vi "运维调试_五参数.vi"() -> ()   [LabVIEW 2016, in "斯坦道仪器.lvlib"]
uses:
  <vilib>/Utility/miscctls.llb/LVPointTypeDef.ctl
  <vilib>/Utility/config.llb/NI_LVConfig.lvlib
panel:
  in  "质控参数设置":bool
  in  "打开串口":bool
  in  "释放串口":bool
  out "多参数横条运行状态":T1(xcontrol)
  in  "数据区":i32(listbox)
  in  "探头选择":u16(ring)=9 items=["氨氮"=3, "水温"=9, "pH值"=10, "溶解氧"=11, "电导率"=12, "浊度"=13, "叶绿素a"=14, "藻密度"=15, "蓝绿藻"=16, "氧化还原电位"=17, "溶解氧%"=18, "盐度"=19]
  in  "测量数据区读取":bool
  in  "测量数据区":i32(listbox)
  in  "状态告警区读取":bool
  in  "状态告警区":i32(listbox)
  in  "读取KB":bool
  in  "写入KB":bool
  out "B":dbl caption="校准值B:"
  out "K":dbl caption="校准值K:"
  in  "校准区探头选择":u16(ring)=9 items=["氨氮"=3, "水温"=9, "pH值"=10, "溶解氧"=11, "电导率"=12, "浊度"=13, "叶绿素a"=14, "藻密度"=15, "蓝绿藻"=16, "氧化还原电位"=17, "溶解氧%"=18, "盐度"=19]
  in  "停止测量(单探)":bool
  in  "启动测量(单探)":bool
  in  "控制命令区探头选择":u16(ring)=9 items=["氨氮"=3, "水温"=9, "pH值"=10, "溶解氧"=11, "电导率"=12, "浊度"=13, "叶绿素a"=14, "藻密度"=15, "蓝绿藻"=16, "氧化还原电位"=17, "溶解氧%"=18, "盐度"=19]
  in  "同步时间":bool
  in  "初始化(清洗)":bool
  in  "停止测量(全部)":bool
  in  "启动测量(全部)":bool
  in  "关键参数区读取":bool
  in  "关键参数区":i32(listbox)
  in  "传感器参数读取":bool
  in  "传感器区":i32(listbox)
  in  "返回":bool
  in  "设置":bool
  out "运行状态":string
  out "开机状态":bool
  in  "停止":bool
  in  "手动启动":bool
  out "集成报警信息":string
  # "控制命令区"
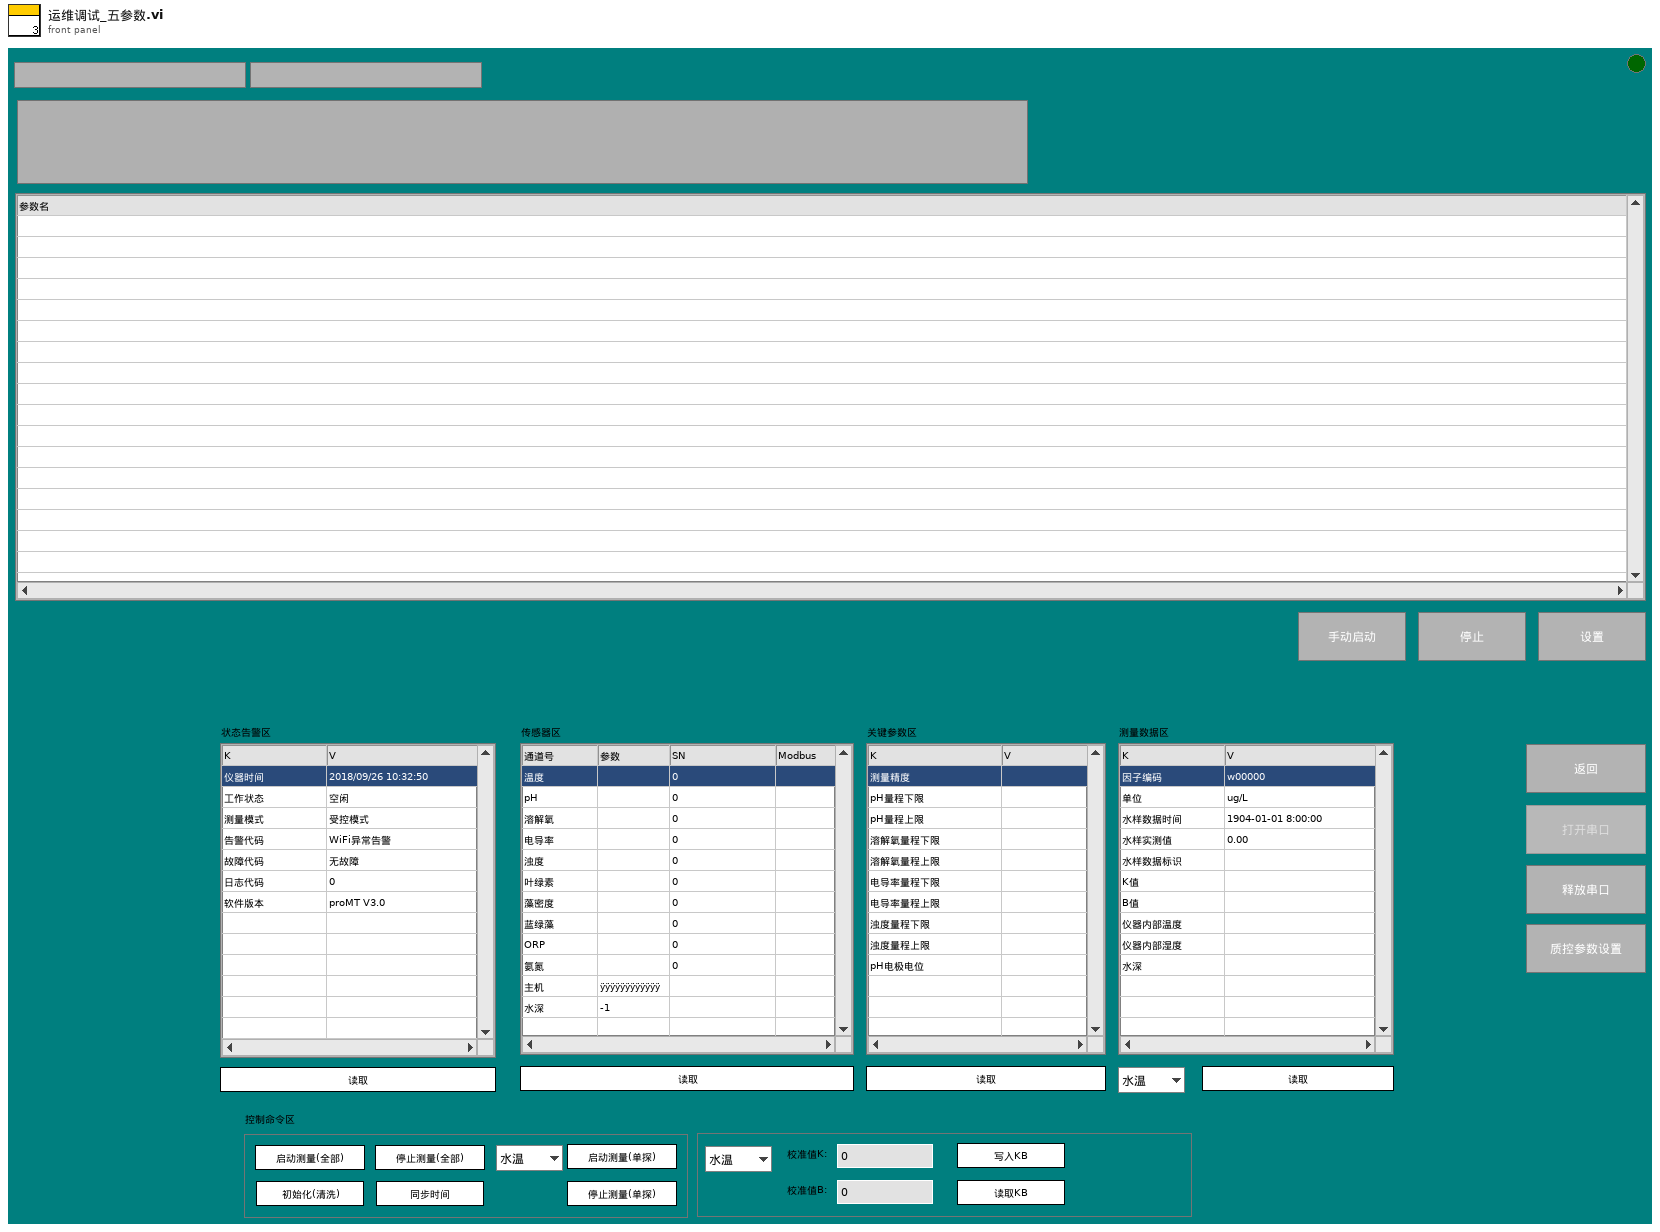
[diagram p1: front panel]
types:
  T1 = cluster{"系统时间":timestamp, "工作状态":u16, "测量模式":u16, "告警代码":enum16{"无告警", "缺试剂告警", "缺水样告警", "缺蒸馏水告警", "缺标液告警", "仪表漏液告警", "标定异常告警", "超量程告警", "加热异常", "低试剂预警", "超上限告警", "超下限告警", "仪表内部其他异常", "滴定异常告警", "电极异常告警", "量程切换告警", "参数设置告警", "PH电极电位异常", "电导率电极异常", "浊度光度异常", "溶解氧电极异常", "溶解氧光强异常", "温度异常告警", "PH异常告警", "溶解氧异常告警", "电导率异常告警", "浊度异常告警", "叶绿素异常告警", "藻密度异常告警", "蓝绿藻异常告警", "ORP异常告警", "氨氮异常告警", "清洁刷异常告警", "SD卡异常告警", "蓝牙异常告警", "Wifi异常告警", "流程异常告警"}, "故障代码":enum16{"无故障", "电机故障", "温度故障", "通讯故障", "滴定故障"}, "日志代码":u16, "软件版本":string}
  T2 = typedef "LVPointTypeDef.ctl" = cluster{"Horizontal":i16, "Vertical":i16}
  T3 = cluster{"时间标识":timestamp, "设备":string, "日志信息":string}
  T4 = enum16{"无告警", "缺试剂告警", "缺水样告警", "缺蒸馏水告警", "缺标液告警", "仪表漏液告警", "标定异常告警", "超量程告警", "加热异常", "低试剂预警", "超上限告警", "超下限告警", "仪表内部其他异常", "滴定异常告警", "电极异常告警", "量程切换告警", "参数设置告警", "PH电极电位异常", "电导率电极异常", "浊度光度异常", "溶解氧电极异常", "溶解氧光强异常", "温度异常告警", "PH异常告警", "溶解氧异常告警", "电导率异常告警", "浊度异常告警", "叶绿素异常告警", "藻密度异常告警", "蓝绿藻异常告警", "ORP异常告警", "氨氮异常告警", "清洁刷异常告警", "SD卡异常告警", "蓝牙异常告警", "Wifi异常告警", "流程异常告警"}
  T5 = cluster{"水温":dbl, "pH":dbl, "DO":dbl, "Cond":dbl, "Turb":dbl, "叶绿素":dbl, "藻密度":dbl, "蓝绿藻":dbl, "ORP":dbl, "NH3N":dbl}
  T6 = cluster{"因子编码":string, "单位":string, "标样参考值":sgl, "水样数据时间":timestamp, "水样实测值":sgl, "水样数据标识":string, "K":sgl, "B":sgl, "T":sgl, "H":sgl, "水深":sgl, "探头温度":sgl}
  T7 = typedef "NI_LVConfig.lvlib/Config Data RefNum.ctl" = refnum<k1>
  T8 = enum8{"Enabled", "Disabled", "Disabled and Grayed Out"}
  T9 = cluster{"测量模式":enum16{"待机", "水样测试", "标样核查", "零点核查", "跨度核查", "空白测试", "平行样测试", "加标回收", "空白校准", "标样校准", "初始化（清洗）"}, "数据标记表":string, "测量时间":dbl}
  T10 = cluster{"水温标准液标准浓度":dbl, "酸碱度标准液标准浓度":dbl, "溶解氧标准液标准浓度":dbl, "电导率标准液标准浓度":dbl, "浊度标准液标准浓度":dbl}
  T11 = cluster{"确定":bool, "水温标准液标准浓度":dbl, "酸碱度标准液标准浓度":dbl, "溶解氧标准液标准浓度":dbl, "电导率标准液标准浓度":dbl, "浊度标准液标准浓度":dbl}
  T12 = enum32{"Bad", "Idle", "Run top level", "Running"}
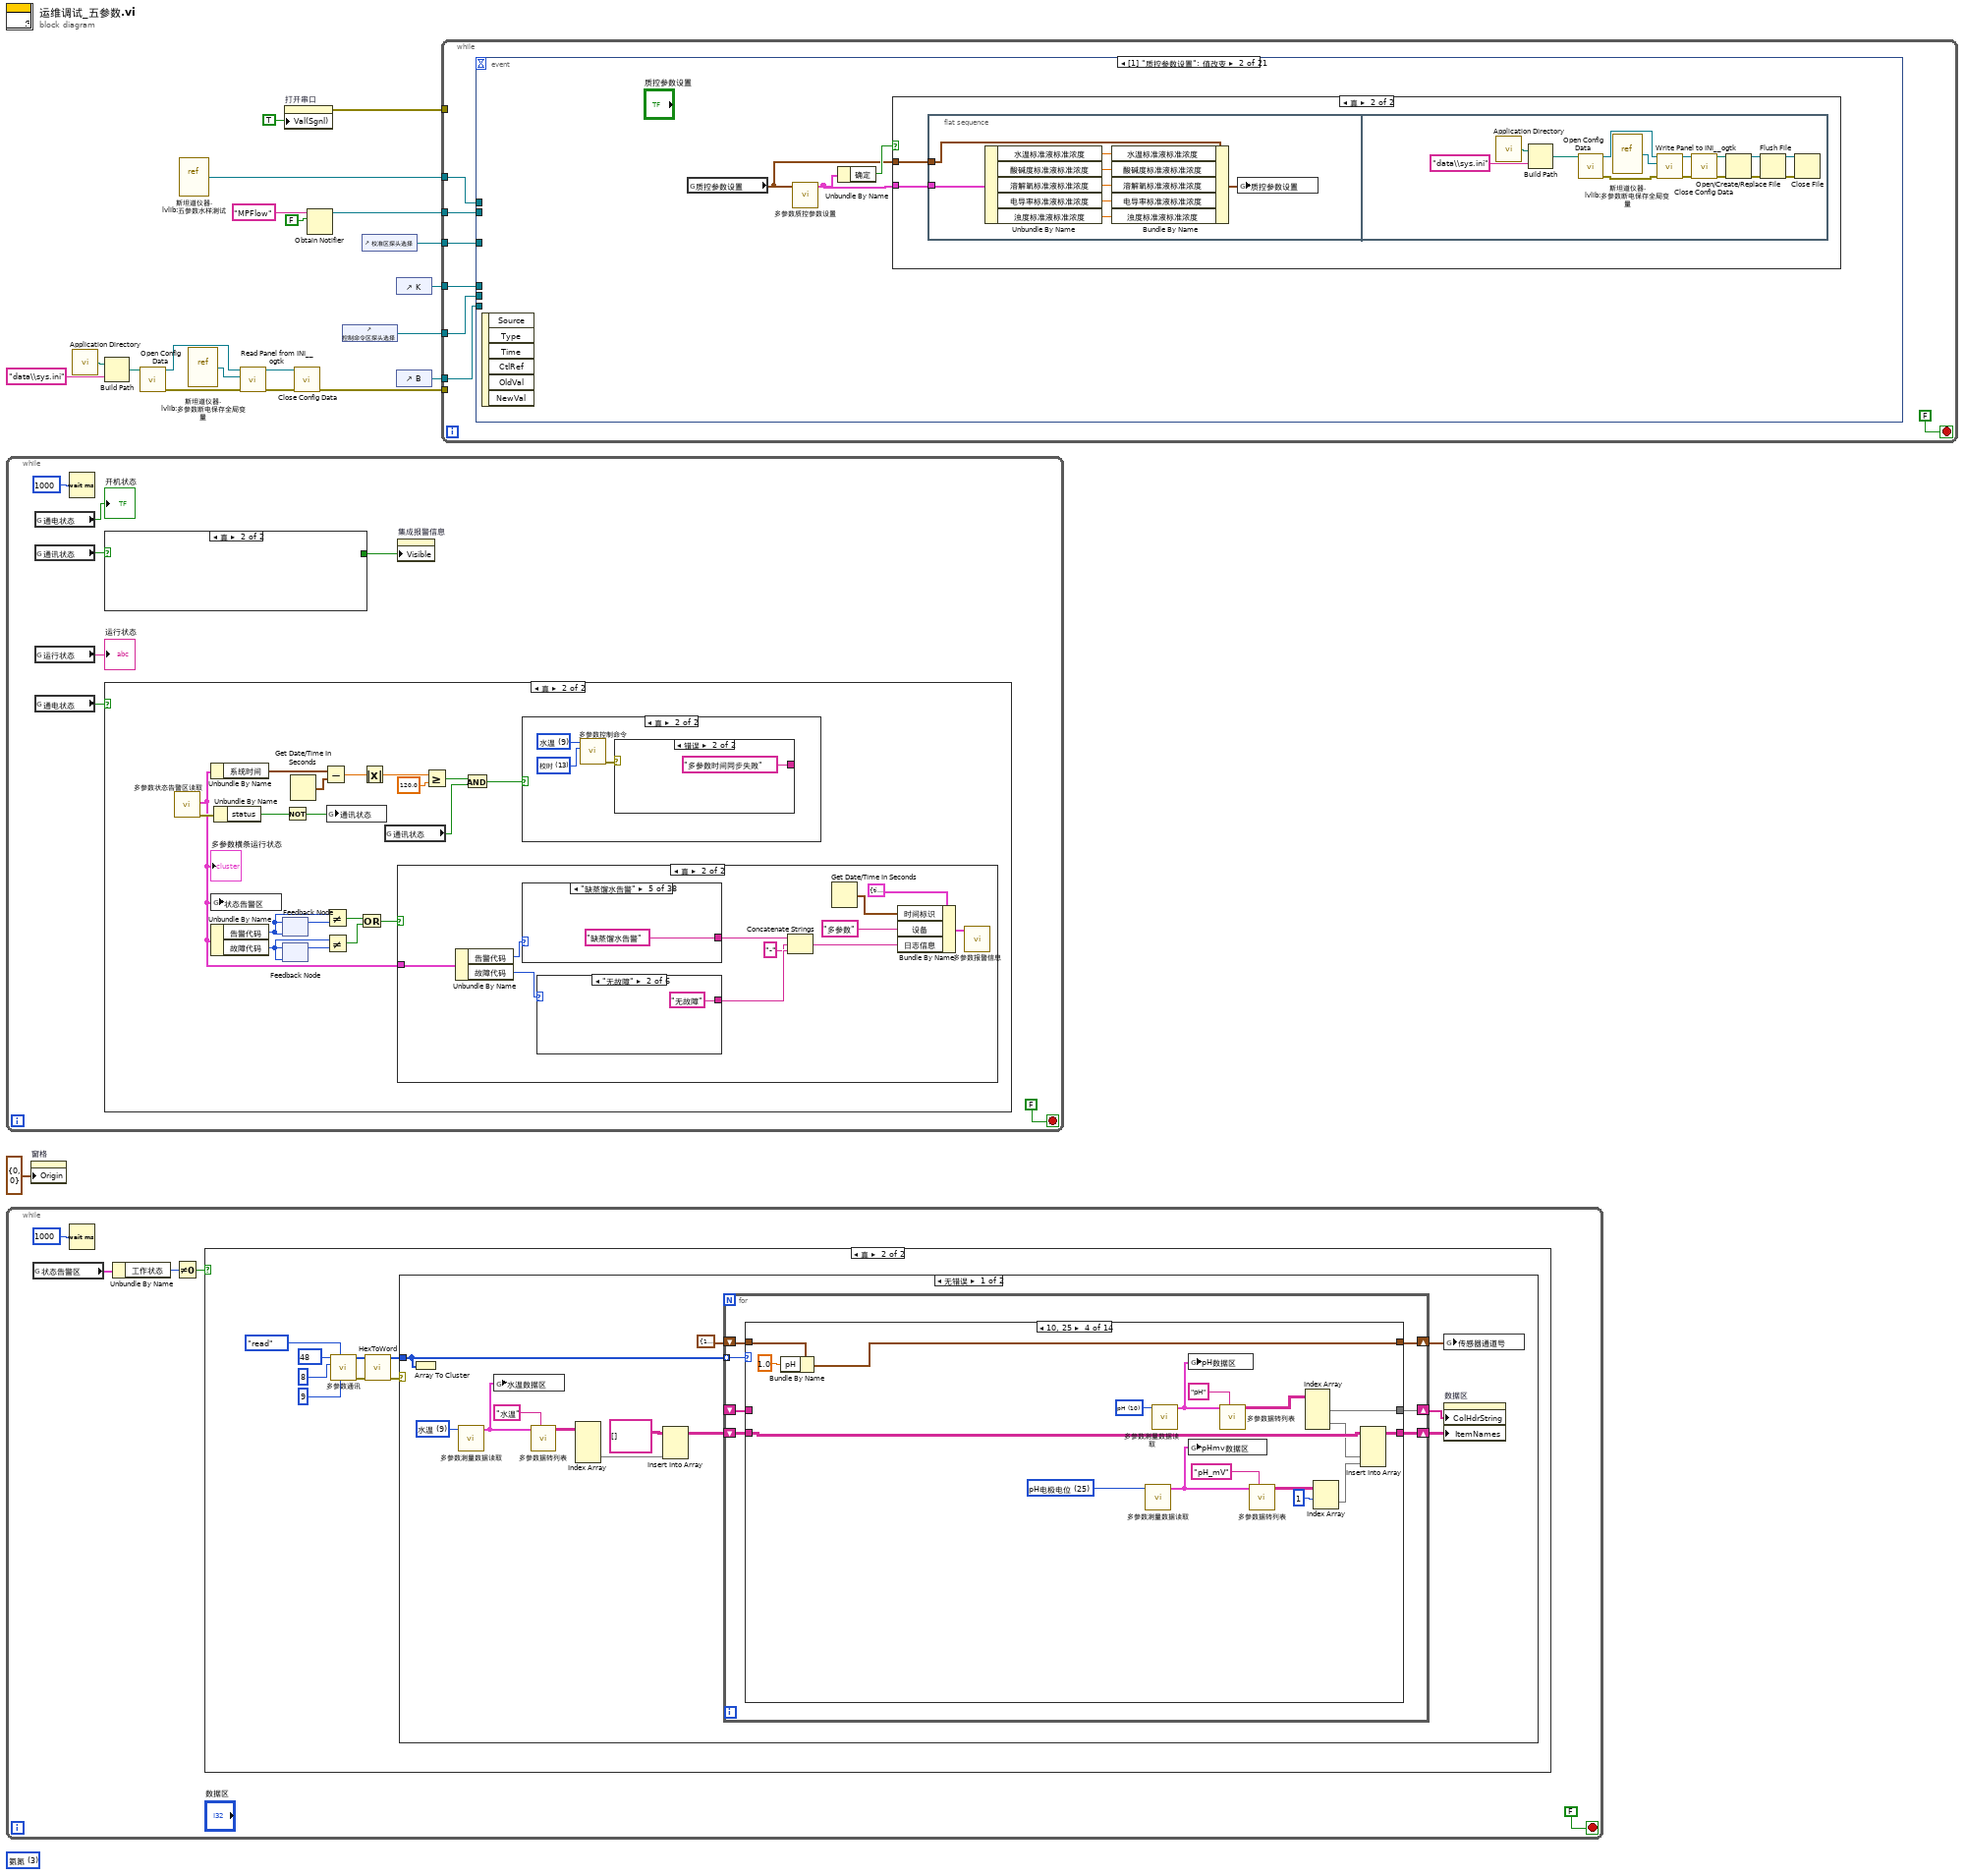
[diagram p0: block diagram]
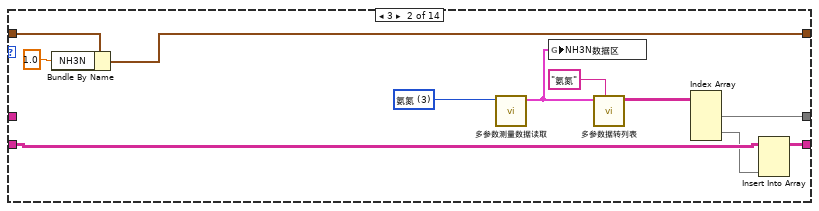
[diagram p4: hidden frame]
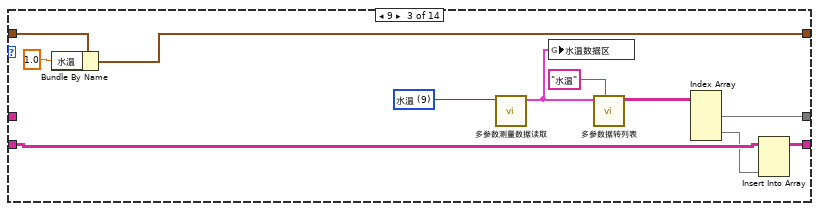
[diagram p5: hidden frame]
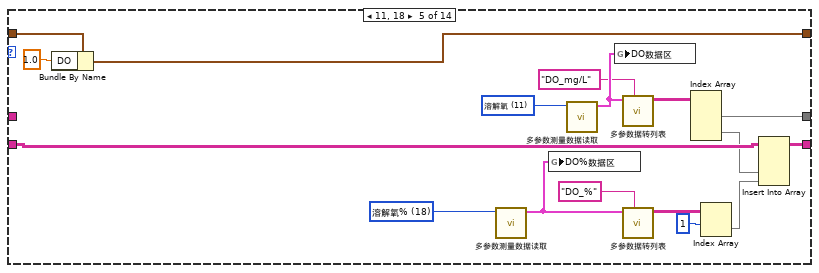
[diagram p6: hidden frame]
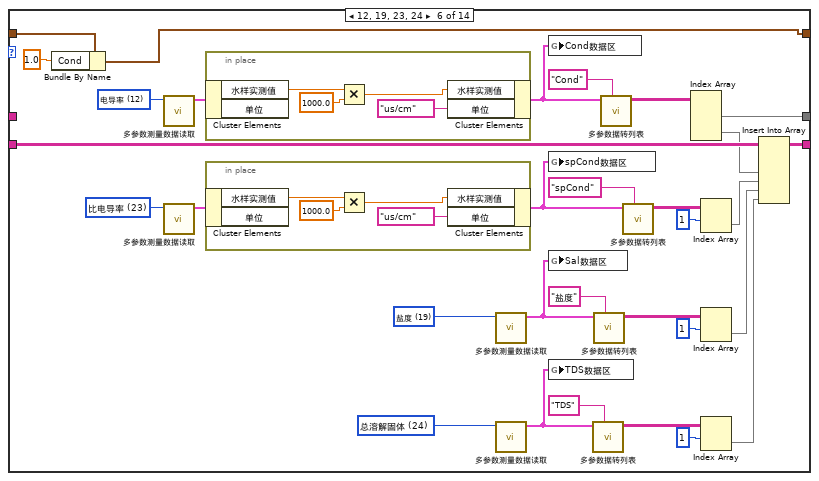
[diagram p7: hidden frame]
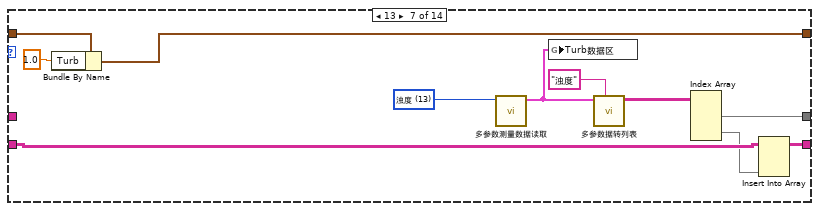
[diagram p8: hidden frame]
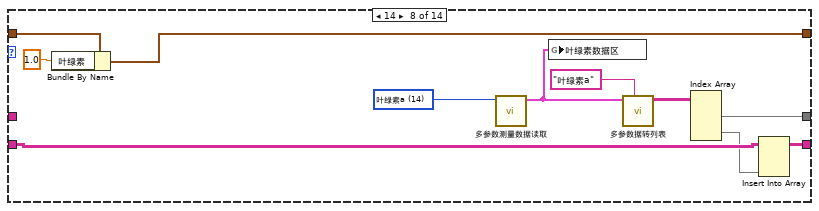
[diagram p9: hidden frame]
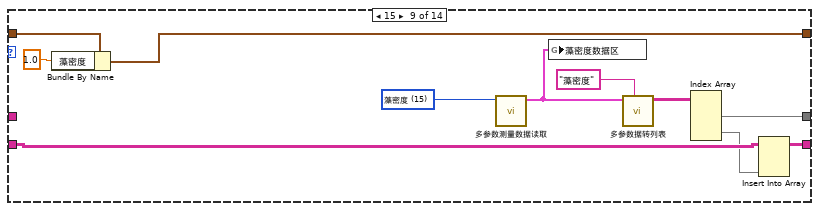
[diagram p10: hidden frame]
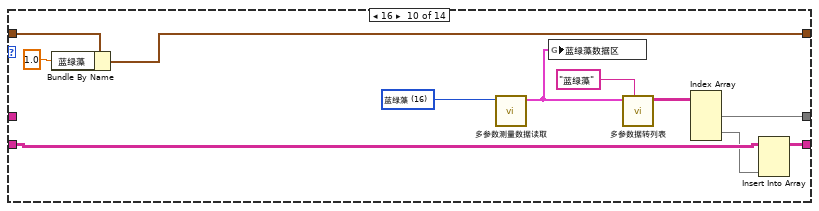
[diagram p11: hidden frame]
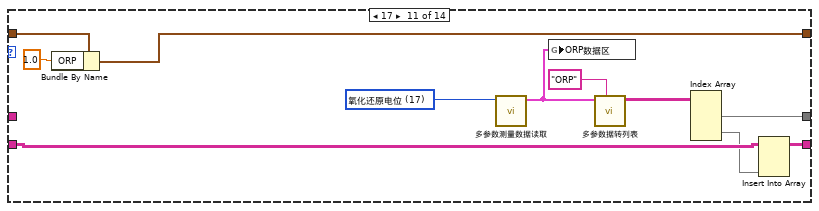
[diagram p12: hidden frame]
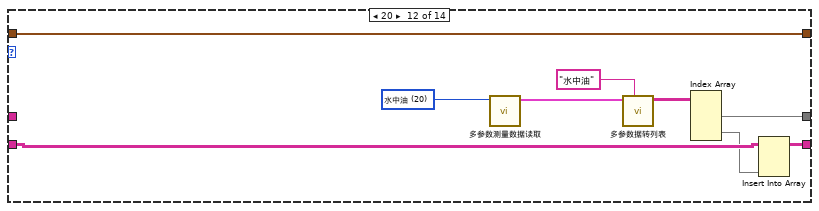
[diagram p13: hidden frame]
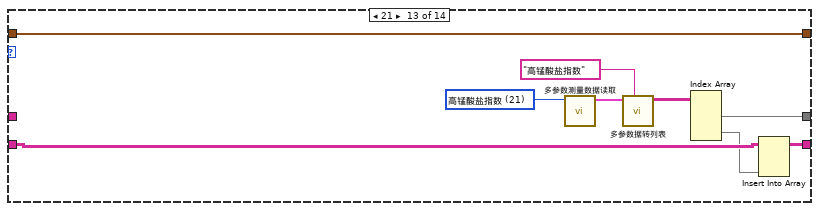
[diagram p14: hidden frame]
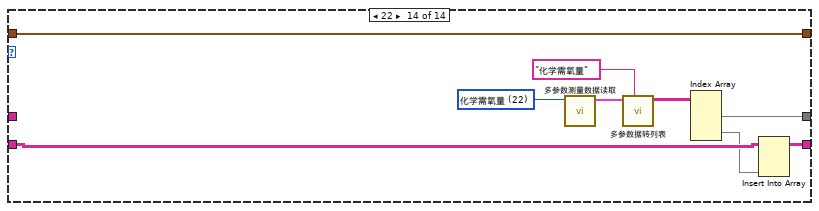
[diagram p15: hidden frame]
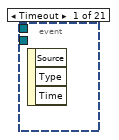
[diagram p17: hidden frame]
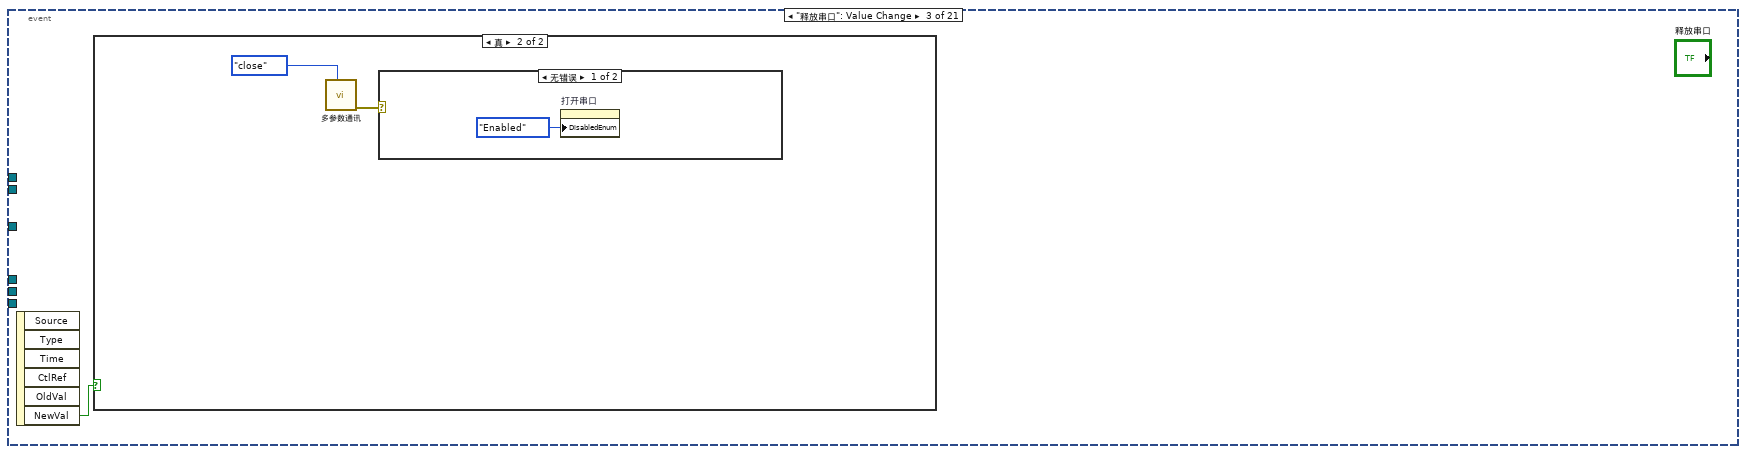
[diagram p19: hidden frame]
diagram:
  (unwired) u16 3 items=["氨氮"=3, "水温"=9, "pH"=10, "溶解氧"=11, "电导率"=12, "浊度"=13, "叶绿素a"=14, "藻密度"=15, "蓝绿藻"=16, "氧化还原电位"=17, "溶解氧%"=18, "盐度"=19, "水中油"=20, "高锰酸盐指数"=21, "化学需氧量"=22, "比电导率"=23, "总溶解固体"=24, "pH电极电位"=25] ("下拉列表")
  n1 = while {
    stop <- FALSE stop-if-true
    n2 = global read "多参数全局变量.vi" "通电状态"() -> (→"开机状态":bool)
    n3 = global read "多参数全局变量.vi" "通讯状态"() -> (w25:bool)
    n4 = global read "多参数全局变量.vi" "运行状态"() -> (→"运行状态":string)
    n5 = global read "多参数全局变量.vi" "通电状态"() -> (w21:bool)
    n6 = Wait (ms)(milliseconds to wait=u32 1000 ("等待时间（毫秒）")) -> ()  [unwired: 1 out]
    n7 = case shown="真" w25 {
      tunnel: [TRUE ("可见") _] -> w24
      frame False {
        "集成报警信息" <- "通讯异常" ("集成报警信息")
      }
      frame True {
      }
    }
    n8 = case shown="真" w21 {
      frame False {
      }
      frame True {
        n9 = call "多参数状态告警区读取.vi"() -> ("error out"=w39:errorcluster, "状态告警块"=w36:T1)  [unwired: 9 in, 1 out]
        "多参数横条运行状态" <- w36
        n10 = Unbundle By Name(w36) -> ("系统时间"=w35:timestamp)
        n11 = global write "多参数全局变量.vi" "状态告警区"(w36) -> ()
        n12 = Unbundle By Name(w36) -> ("告警代码"=w45:T4, "故障代码"=w43:enum16{"无故障", "电机故障", "温度故障", "通讯故障", "滴定故障"})
        n13 = Unbundle By Name(w39) -> ("status"=w38:bool)
        n14 = feedback #1(w45) -> (w46:T4)
        n15 = feedback-in #1(w45) -> ()
        n16 = feedback #2(w43) -> (w44:enum16{"无故障", "电机故障", "温度故障", "通讯故障", "滴定故障"})
        n17 = feedback-in #2(w43) -> ()
        n18 = Not(x=w38) -> (.not. x?=w37:bool)
        n19 = Get Date/Time In Seconds() -> (seconds since 1Jan1904=w34:timestamp)
        n20 = Subtract(x=w35, y=w34) -> (x-y=w33:dbl)
        n21 = Not Equal?(x=w45, y=w46) -> (x != y?=w41:bool)
        n22 = Not Equal?(x=w43, y=w44) -> (x != y?=w42:bool)
        n23 = global write "多参数全局变量.vi" "通讯状态"(w37) -> ()
        n24 = Or(x=w41, y=w42) -> (x .or. y?=w40:bool)
        n25 = Absolute Value(x=w33) -> (abs(x)=w32:dbl)
        n26 = global read "多参数全局变量.vi" "通讯状态"() -> (w28:bool)
        n27 = case shown="真" w40 {
          tunnel: w36 -> [_ w62]
          frame False {
          }
          frame True {
            n28 = Unbundle By Name(w62) -> ("告警代码"=w61:T4, "故障代码"=w60:enum16{"无故障", "电机故障", "温度故障", "通讯故障", "滴定故障"})
            n29 = case shown="\"缺蒸馏水告警\"" w61 {
              selector: w61 -> [w73 _ _ _ _ _ _ _ _ _ _ _ _ _ _ _ _ _ _ _ _ _ _ _ _ _ _ _ _ _ _ _ _ _ _ _ _ _]
              tunnel: [w72 "无告警" "缺试剂告警" "缺水样告警" "缺蒸馏水告警" "缺标液告警" "仪表漏液告警" "标定异常告警" "超量程告警" "加热异常" "低试剂预警" "超上限告警" "超下限告警" "仪表内部其他异常" "滴定异常告警" "电极异常告警" "量程切换告警" "参数设置告警" "PH电极电位异常" "电导率电极异常" "浊度光度异常" "溶解氧电极异常" "溶解氧光强异常" "温度异常告警" "PH异常告警" "溶解氧异常告警" "电导率异常告警" "浊度异常告警" "叶绿素异常告警" "藻密度异常告警" "蓝绿藻异常告警" "ORP异常告警" "氨氮异常告警" "清洁刷异常告警" "SD卡异常告警" "蓝牙异常告警" "WiFi异常告警" "流程异常告警"] -> w59
              frame Default {
                n30 = Format Into String(format string="%d" ("格式字符串"), initial string="未知" ("工作状态"), w73) -> (resulting string=w72:string)  [unwired: 1 in, 1 out]
              }
              frame "无告警" {
              }
              frame "缺试剂告警" {
              }
              frame "缺水样告警" {
              }
              frame "缺蒸馏水告警" {
              }
              frame "缺标液告警" {
              }
              frame "仪表漏液告警" {
              }
              frame "标定异常告警" {
              }
              frame "超量程告警" {
              }
              frame "加热异常" {
              }
              frame "低试剂预警" {
              }
              frame "超上限告警" {
              }
              frame "超下限告警" {
              }
              frame "仪表内部其他异常" {
              }
              frame "滴定异常告警" {
              }
              frame "电极异常告警" {
              }
              frame "量程切换告警" {
              }
              frame "参数设置告警" {
              }
              frame "PH电极电位异常" {
              }
              frame "电导率电极异常" {
              }
              frame "浊度光度异常" {
              }
              frame "溶解氧电极异常" {
              }
              frame "溶解氧光强异常" {
              }
              frame "温度异常告警" {
              }
              frame "PH异常告警" {
              }
              frame "溶解氧异常告警" {
              }
              frame "电导率异常告警" {
              }
              frame "浊度异常告警" {
              }
              frame "叶绿素异常告警" {
              }
              frame "藻密度异常告警" {
              }
              frame "蓝绿藻异常告警" {
              }
              frame "ORP异常告警" {
              }
              frame "氨氮异常告警" {
              }
              frame "清洁刷异常告警" {
              }
              frame "SD卡异常告警" {
              }
              frame "蓝牙异常告警" {
              }
              frame "Wifi异常告警" {
              }
              frame "流程异常告警" {
              }
            }
            n31 = case shown="\"无故障\"" w60 {
              selector: w60 -> [w64 _ _ _ _ _]
              tunnel: [w63 "无故障" "电机故障" "温度故障" "通讯故障" "滴定故障"] -> w58
              frame Default {
                n32 = Format Into String(format string="%d" ("格式字符串"), initial string="未知" ("工作状态"), w64) -> (resulting string=w63:string)  [unwired: 1 in, 1 out]
              }
              frame "无故障" {
              }
              frame "电机故障" {
              }
              frame "温度故障" {
              }
              frame "通讯故障" {
              }
              frame "滴定故障" {
              }
            }
            n33 = Concatenate Strings(w59, "-" ("字符串"), w58) -> (w54:string)
            n34 = Get Date/Time In Seconds() -> (seconds since 1Jan1904=w53:timestamp)
            n35 = Bundle By Name(cluster=T3 {"时间标识"=timestamp(0 s since 1904-01-01), "设备"="", "日志信息"=""} ("data in"), "时间标识"=w53, "设备"="多参数", "日志信息"=w54) -> (w55:T3)
            n36 = call "多参数报警信息.vi"("data in"=w55) -> ()  [unwired: 10 in, 1 out]
          }
        }
        n37 = Greater Or Equal?(x=w32, y=120.0) -> (x >= y?=w31:bool)
        n38 = And(x=w31, y=w28) -> (x .and. y?=w29:bool)
        n39 = case shown="真" w29 {
          frame False {
          }
          frame True {
            w47 = u16 13 items=["启动测量（全部）"=1, "初始化（清洗）"=10, "停止测量（全部）"=11, "校时"=13, "启动测量（单个传感器）"=19, "停止测量（单个传感器）"=20] ("控制命令")
            w48 = u16 9 items=["氨氮"=3, "水温"=9, "pH值"=10, "溶解氧"=11, "电导率"=12, "浊度"=13, "叶绿素a"=14, "藻密度"=15, "蓝绿藻"=16, "氧化还原电位"=17, "溶解氧%"=18, "盐度"=19] ("站号")
            n40 = call "多参数控制命令.vi"("控制命令"=w47, "站号"=w48) -> ("error out"=w49:errorcluster)  [unwired: 9 in]
            n41 = case shown="错误" w49 {
              tunnel: ["多参数时间同步成功" ("消息") "多参数时间同步失败" ("消息")] -> _
              frame No Error {
              }
              frame Error {
              }
            }
          }
        }
      }
    }
    n42 = property on="集成报警信息" class="Str"("Visible"=w24) -> ()  [unwired: 2 in, 2 out]
  }
  n43 = while {
    stop <- FALSE stop-if-true
    n44 = global read "多参数全局变量.vi" "状态告警区"() -> (w117:T1)
    n45 = Wait (ms)(milliseconds to wait=u32 1000 ("等待时间（毫秒）")) -> ()  [unwired: 1 out]
    n46 = Unbundle By Name(w117) -> ("工作状态"=w116:u16)
    n47 = Not Equal To 0?(x=w116) -> (x != 0?=w115:bool)
    n48 = case shown="真" w115 {
      frame False {
      }
      frame True {
        n49 = call "多参数通讯.vi"("Slave ID"=u8 9, "STEP"=enum16{"open", "read", "write", "close"}."read", "quantity"=u16 8, "starting address"=u16 48) -> ("error out"=w122:errorcluster, "Registers"=w123:u16[])  [unwired: 5 in, 1 out]
        n50 = call "HexToWord.vi"("数组"=w123) -> ("WORD"=w126:u16[])  [unwired: 10 in]
        n51 = case shown="无错误" w122 {
          tunnel: w126 -> [w138 _]
          frame No Error {
            w135 = u16 9 items=["氨氮"=3, "水温"=9, "pH"=10, "溶解氧"=11, "电导率"=12, "浊度"=13, "叶绿素a"=14, "藻密度"=15, "蓝绿藻"=16, "氧化还原电位"=17, "溶解氧%"=18, "盐度"=19, "水中油"=20, "高锰酸盐指数"=21, "化学需氧量"=22, "比电导率"=23, "总溶解固体"=24, "pH电极电位"=25] ("下拉列表")
            n52 = Array To Cluster(array=w138) -> ()  [unwired: 1 out]
            n53 = call "多参数测量数据读取.vi"("探头选择"=w135) -> ("测量数据块"=w130:T6)  [unwired: 8 in, 2 out]
            n54 = global write "多参数全局变量.vi" "水温数据区"(w130) -> ()
            n55 = call "多参数据转列表.vi"("参数名"="水温", "测量数据块"=w130) -> ("添加的数组"=w128:string[][])  [unwired: 9 in]
            n56 = Index Array(array=w128) -> (element #2=w127:string[])  [unwired: 4 in, 1 out]
            n57 = Insert Into Array(array=string[][] [] ("子数组"), new element=w127) -> (w133:string[][])  [unwired: 2 in]
            n58 = for {
              tunnel: w138 -> [w145] mode=indexing
              shift-right: [w143] -> w136
              shift-left: w133 -> [w144]
              shift-right: [w142] -> w137
              shift-left: _ -> [w141]
              shift-right: [w140] -> w131
              shift-left: T5 {"水温"=1.0, "pH"=0.0, "DO"=0.0, "Cond"=0.0, "Turb"=0.0, "叶绿素"=0.0, "藻密度"=0.0, "蓝绿藻"=0.0, "ORP"=0.0, "NH3N"=0.0} ("传感器通道号") -> [w139]
              n59 = case shown="10, 25" w145 {
                tunnel: w144 -> [w148 w158 w169 w186 w203 w234 w253 w264 w275 w286 w297 w306 w315 w324]
                tunnel: [w148 w157 w168 w185 w202 w233 w252 w263 w274 w285 w296 w305 w314 w323] -> w143
                tunnel: [w147 w150 w161 w178 w195 w224 w246 w256 w269 w279 w290 w300 w309 w318] -> w142
                tunnel: w141 -> [w147 _ _ _ _ _ _ _ _ _ _ _ _ _]
                tunnel: [w146 w154 w165 w181 w199 w227 w249 w260 w271 w282 w293 w304 w313 w322] -> w140
                tunnel: w139 -> [w146 w156 w167 w183 w201 w228 w250 w261 w272 w283 w294 w304 w313 w322]
                frame 0, Default {
                }
                frame 3 {
                  w159 = u16 3 items=["氨氮"=3, "水温"=9, "pH"=10, "溶解氧"=11, "电导率"=12, "浊度"=13, "叶绿素a"=14, "藻密度"=15, "蓝绿藻"=16, "氧化还原电位"=17, "溶解氧%"=18, "盐度"=19, "水中油"=20, "高锰酸盐指数"=21, "化学需氧量"=22, "比电导率"=23, "总溶解固体"=24, "pH电极电位"=25] ("下拉列表")
                  n60 = Bundle By Name(cluster=w156, "NH3N"=1.0) -> (w154:T5)
                  n61 = call "多参数测量数据读取.vi"("探头选择"=w159) -> ("测量数据块"=w153:T6)  [unwired: 8 in, 2 out]
                  n62 = global write "多参数全局变量.vi" "NH3N数据区"(w153) -> ()
                  n63 = call "多参数据转列表.vi"("参数名"="氨氮", "测量数据块"=w153) -> ("添加的数组"=w152:string[][])  [unwired: 9 in]
                  n64 = Index Array(array=w152) -> (element #1=w150:string[], element #2=w149:string[])  [unwired: 4 in]
                  n65 = Insert Into Array(array=w158, new element=w149) -> (w157:string[][])  [unwired: 2 in]
                }
                frame 9 {
                  w170 = u16 9 items=["氨氮"=3, "水温"=9, "pH"=10, "溶解氧"=11, "电导率"=12, "浊度"=13, "叶绿素a"=14, "藻密度"=15, "蓝绿藻"=16, "氧化还原电位"=17, "溶解氧%"=18, "盐度"=19, "水中油"=20, "高锰酸盐指数"=21, "化学需氧量"=22, "比电导率"=23, "总溶解固体"=24, "pH电极电位"=25] ("下拉列表")
                  n66 = Bundle By Name(cluster=w167, "水温"=1.0) -> (w165:T5)
                  n67 = call "多参数测量数据读取.vi"("探头选择"=w170) -> ("测量数据块"=w164:T6)  [unwired: 8 in, 2 out]
                  n68 = global write "多参数全局变量.vi" "水温数据区"(w164) -> ()
                  n69 = call "多参数据转列表.vi"("参数名"="水温", "测量数据块"=w164) -> ("添加的数组"=w163:string[][])  [unwired: 9 in]
                  n70 = Index Array(array=w163) -> (element #1=w161:string[], element #2=w160:string[])  [unwired: 4 in]
                  n71 = Insert Into Array(array=w169, new element=w160) -> (w168:string[][])  [unwired: 2 in]
                }
                frame 10, 25 {
                  w184 = u16 25 items=["氨氮"=3, "水温"=9, "pH"=10, "溶解氧"=11, "电导率"=12, "浊度"=13, "叶绿素a"=14, "藻密度"=15, "蓝绿藻"=16, "氧化还原电位"=17, "溶解氧%"=18, "盐度"=19, "水中油"=20, "高锰酸盐指数"=21, "化学需氧量"=22, "比电导率"=23, "总溶解固体"=24, "pH电极电位"=25] ("下拉列表")
                  w187 = u16 10 items=["氨氮"=3, "水温"=9, "pH"=10, "溶解氧"=11, "电导率"=12, "浊度"=13, "叶绿素a"=14, "藻密度"=15, "蓝绿藻"=16, "氧化还原电位"=17, "溶解氧%"=18, "盐度"=19, "水中油"=20, "高锰酸盐指数"=21, "化学需氧量"=22, "比电导率"=23, "总溶解固体"=24, "pH电极电位"=25] ("下拉列表")
                  n72 = Bundle By Name(cluster=w183, "pH"=1.0) -> (w181:T5)
                  n73 = call "多参数测量数据读取.vi"("探头选择"=w184) -> ("测量数据块"=w174:T6)  [unwired: 8 in, 2 out]
                  n74 = call "多参数测量数据读取.vi"("探头选择"=w187) -> ("测量数据块"=w180:T6)  [unwired: 8 in, 2 out]
                  n75 = global write "多参数全局变量.vi" "pH数据区"(w180) -> ()
                  n76 = global write "多参数全局变量.vi" "pHmv数据区"(w174) -> ()
                  n77 = call "多参数据转列表.vi"("参数名"="pH", "测量数据块"=w180) -> ("添加的数组"=w179:string[][])  [unwired: 9 in]
                  n78 = call "多参数据转列表.vi"("参数名"="pH_mV", "测量数据块"=w174) -> ("添加的数组"=w173:string[][])  [unwired: 9 in]
                  n79 = Index Array(array=w179) -> (element #1=w178:string[], element #2=w177:string[])  [unwired: 4 in]
                  n80 = Index Array(array=w173, index (row)=1 ("禁用的索引 (列)")) -> (element=w176:string[])  [unwired: 1 in]
                  n81 = Insert Into Array(array=w186, new element #1=w177, new element #2=w176) -> (w185:string[][])  [unwired: 2 in]
                }
                frame 11, 18 {
                  w193 = u16 18 items=["氨氮"=3, "水温"=9, "pH"=10, "溶解氧"=11, "电导率"=12, "浊度"=13, "叶绿素a"=14, "藻密度"=15, "蓝绿藻"=16, "氧化还原电位"=17, "溶解氧%"=18, "盐度"=19, "水中油"=20, "高锰酸盐指数"=21, "化学需氧量"=22, "比电导率"=23, "总溶解固体"=24, "pH电极电位"=25] ("下拉列表")
                  w204 = u16 11 items=["氨氮"=3, "水温"=9, "pH"=10, "溶解氧"=11, "电导率"=12, "浊度"=13, "叶绿素a"=14, "藻密度"=15, "蓝绿藻"=16, "氧化还原电位"=17, "溶解氧%"=18, "盐度"=19, "水中油"=20, "高锰酸盐指数"=21, "化学需氧量"=22, "比电导率"=23, "总溶解固体"=24, "pH电极电位"=25] ("下拉列表")
                  n82 = Bundle By Name(cluster=w201, "DO"=1.0) -> (w199:T5)
                  n83 = call "多参数测量数据读取.vi"("探头选择"=w193) -> ("测量数据块"=w192:T6)  [unwired: 8 in, 2 out]
                  n84 = global write "多参数全局变量.vi" "DO%数据区"(w192) -> ()
                  n85 = call "多参数测量数据读取.vi"("探头选择"=w204) -> ("测量数据块"=w198:T6)  [unwired: 8 in, 2 out]
                  n86 = global write "多参数全局变量.vi" "DO数据区"(w198) -> ()
                  n87 = call "多参数据转列表.vi"("参数名"="DO_mg/L", "测量数据块"=w198) -> ("添加的数组"=w196:string[][])  [unwired: 9 in]
                  n88 = call "多参数据转列表.vi"("参数名"="DO_%", "测量数据块"=w192) -> ("添加的数组"=w190:string[][])  [unwired: 9 in]
                  n89 = Index Array(array=w196) -> (element #1=w195:string[], element #2=w194:string[])  [unwired: 4 in]
                  n90 = Index Array(array=w190, index (row)=1 ("禁用的索引 (列)")) -> (element=w189:string[])  [unwired: 1 in]
                  n91 = Insert Into Array(array=w203, new element #1=w194, new element #2=w189) -> (w202:string[][])  [unwired: 2 in]
                }
                frame 12, 19, 23, 24 {
                  w230 = u16 24 items=["氨氮"=3, "水温"=9, "pH"=10, "溶解氧"=11, "电导率"=12, "浊度"=13, "叶绿素a"=14, "藻密度"=15, "蓝绿藻"=16, "氧化还原电位"=17, "溶解氧%"=18, "盐度"=19, "水中油"=20, "高锰酸盐指数"=21, "化学需氧量"=22, "比电导率"=23, "总溶解固体"=24, "pH电极电位"=25] ("下拉列表")
                  w231 = u16 19 items=["氨氮"=3, "水温"=9, "pH"=10, "溶解氧"=11, "电导率"=12, "浊度"=13, "叶绿素a"=14, "藻密度"=15, "蓝绿藻"=16, "氧化还原电位"=17, "溶解氧%"=18, "盐度"=19, "水中油"=20, "高锰酸盐指数"=21, "化学需氧量"=22, "比电导率"=23, "总溶解固体"=24, "pH电极电位"=25] ("下拉列表")
                  w232 = u16 23 items=["氨氮"=3, "水温"=9, "pH"=10, "溶解氧"=11, "电导率"=12, "浊度"=13, "叶绿素a"=14, "藻密度"=15, "蓝绿藻"=16, "氧化还原电位"=17, "溶解氧%"=18, "盐度"=19, "水中油"=20, "高锰酸盐指数"=21, "化学需氧量"=22, "比电导率"=23, "总溶解固体"=24, "pH电极电位"=25] ("下拉列表")
                  w235 = u16 12 items=["氨氮"=3, "水温"=9, "pH"=10, "溶解氧"=11, "电导率"=12, "浊度"=13, "叶绿素a"=14, "藻密度"=15, "蓝绿藻"=16, "氧化还原电位"=17, "溶解氧%"=18, "盐度"=19, "水中油"=20, "高锰酸盐指数"=21, "化学需氧量"=22, "比电导率"=23, "总溶解固体"=24, "pH电极电位"=25] ("下拉列表")
                  n92 = Bundle By Name(cluster=w228, "Cond"=1.0 ("DO")) -> (w227:T5)
                  n93 = call "多参数测量数据读取.vi"("探头选择"=w235) -> ("测量数据块"=w211:T6)  [unwired: 8 in, 2 out]
                  n94 = call "多参数测量数据读取.vi"("探头选择"=w232) -> ("测量数据块"=w209:T6)  [unwired: 8 in, 2 out]
                  n95 = in-place {
                    n96 = in-place-cluster #3(w211) -> ("水样实测值"=w242:sgl)  [unwired: 1 out]
                    n97 = Multiply(x=w242, y=sgl 1000.0) -> (x*y=w240:sgl)
                    n98 = in-place-cluster #3("水样实测值"=w240, "单位"="us/cm") -> (w210:T6)
                  }
                  n99 = in-place {
                    n100 = in-place-cluster #4(w209) -> ("水样实测值"=w238:sgl)  [unwired: 1 out]
                    n101 = Multiply(x=w238, y=sgl 1000.0) -> (x*y=w236:sgl)
                    n102 = in-place-cluster #4("水样实测值"=w236, "单位"="us/cm") -> (w208:T6)
                  }
                  n103 = call "多参数测量数据读取.vi"("探头选择"=w231) -> ("测量数据块"=w218:T6)  [unwired: 8 in, 2 out]
                  n104 = call "多参数测量数据读取.vi"("探头选择"=w230) -> ("测量数据块"=w214:T6)  [unwired: 8 in, 2 out]
                  n105 = global write "多参数全局变量.vi" "Cond数据区"(w210) -> ()
                  n106 = global write "多参数全局变量.vi" "spCond数据区"(w208) -> ()
                  n107 = global write "多参数全局变量.vi" "Sal数据区"(w218) -> ()
                  n108 = global write "多参数全局变量.vi" "TDS数据区"(w214) -> ()
                  n109 = call "多参数据转列表.vi"("参数名"="TDS", "测量数据块"=w214) -> ("添加的数组"=w213:string[][])  [unwired: 9 in]
                  n110 = call "多参数据转列表.vi"("参数名"="盐度", "测量数据块"=w218) -> ("添加的数组"=w217:string[][])  [unwired: 9 in]
                  n111 = call "多参数据转列表.vi"("参数名"="Cond", "测量数据块"=w210) -> ("添加的数组"=w225:string[][])  [unwired: 9 in]
                  n112 = call "多参数据转列表.vi"("参数名"="spCond", "测量数据块"=w208) -> ("添加的数组"=w221:string[][])  [unwired: 9 in]
                  n113 = Index Array(array=w225) -> (element #1=w224:string[], element #2=w223:string[])  [unwired: 4 in]
                  n114 = Index Array(array=w221, index (row)=1 ("禁用的索引 (列)")) -> (element=w220:string[])  [unwired: 1 in]
                  n115 = Index Array(array=w217, index (row)=1 ("禁用的索引 (列)")) -> (element=w216:string[])  [unwired: 1 in]
                  n116 = Index Array(array=w213, index (row)=1 ("禁用的索引 (列)")) -> (element=w212:string[])  [unwired: 1 in]
                  n117 = Insert Into Array(array=w234, new element #1=w223, new element #2=w220, new element #3=w216, new element #4=w212) -> (w233:string[][])  [unwired: 2 in]
                }
                frame 13 {
                  w254 = u16 13 items=["氨氮"=3, "水温"=9, "pH"=10, "溶解氧"=11, "电导率"=12, "浊度"=13, "叶绿素a"=14, "藻密度"=15, "蓝绿藻"=16, "氧化还原电位"=17, "溶解氧%"=18, "盐度"=19, "水中油"=20, "高锰酸盐指数"=21, "化学需氧量"=22, "比电导率"=23, "总溶解固体"=24, "pH电极电位"=25] ("下拉列表")
                  n118 = Bundle By Name(cluster=w250, "Turb"=1.0 ("DO")) -> (w249:T5)
                  n119 = call "多参数测量数据读取.vi"("探头选择"=w254) -> ("测量数据块"=w244:T6)  [unwired: 8 in, 2 out]
                  n120 = global write "多参数全局变量.vi" "Turb数据区"(w244) -> ()
                  n121 = call "多参数据转列表.vi"("参数名"="浊度", "测量数据块"=w244) -> ("添加的数组"=w247:string[][])  [unwired: 9 in]
                  n122 = Index Array(array=w247) -> (element #1=w246:string[], element #2=w245:string[])  [unwired: 4 in]
                  n123 = Insert Into Array(array=w253, new element=w245) -> (w252:string[][])  [unwired: 2 in]
                }
                frame 14 {
                  w265 = u16 14 items=["氨氮"=3, "水温"=9, "pH"=10, "溶解氧"=11, "电导率"=12, "浊度"=13, "叶绿素a"=14, "藻密度"=15, "蓝绿藻"=16, "氧化还原电位"=17, "溶解氧%"=18, "盐度"=19, "水中油"=20, "高锰酸盐指数"=21, "化学需氧量"=22, "比电导率"=23, "总溶解固体"=24, "pH电极电位"=25] ("下拉列表")
                  n124 = Bundle By Name(cluster=w261, "叶绿素"=1.0 ("DO")) -> (w260:T5)
                  n125 = call "多参数测量数据读取.vi"("探头选择"=w265) -> ("测量数据块"=w259:T6)  [unwired: 8 in, 2 out]
                  n126 = global write "多参数全局变量.vi" "叶绿素数据区"(w259) -> ()
                  n127 = call "多参数据转列表.vi"("参数名"="叶绿素a", "测量数据块"=w259) -> ("添加的数组"=w257:string[][])  [unwired: 9 in]
                  n128 = Index Array(array=w257) -> (element #1=w256:string[], element #2=w255:string[])  [unwired: 4 in]
                  n129 = Insert Into Array(array=w264, new element=w255) -> (w263:string[][])  [unwired: 2 in]
                }
                frame 15 {
                  w276 = u16 15 items=["氨氮"=3, "水温"=9, "pH"=10, "溶解氧"=11, "电导率"=12, "浊度"=13, "叶绿素a"=14, "藻密度"=15, "蓝绿藻"=16, "氧化还原电位"=17, "溶解氧%"=18, "盐度"=19, "水中油"=20, "高锰酸盐指数"=21, "化学需氧量"=22, "比电导率"=23, "总溶解固体"=24, "pH电极电位"=25] ("下拉列表")
                  n130 = Bundle By Name(cluster=w272, "藻密度"=1.0 ("DO")) -> (w271:T5)
                  n131 = call "多参数测量数据读取.vi"("探头选择"=w276) -> ("测量数据块"=w268:T6)  [unwired: 8 in, 2 out]
                  n132 = global write "多参数全局变量.vi" "藻密度数据区"(w268) -> ()
                  n133 = call "多参数据转列表.vi"("参数名"="藻密度", "测量数据块"=w268) -> ("添加的数组"=w270:string[][])  [unwired: 9 in]
                  n134 = Index Array(array=w270) -> (element #1=w269:string[], element #2=w267:string[])  [unwired: 4 in]
                  n135 = Insert Into Array(array=w275, new element=w267) -> (w274:string[][])  [unwired: 2 in]
                }
                frame 16 {
                  w287 = u16 16 items=["氨氮"=3, "水温"=9, "pH"=10, "溶解氧"=11, "电导率"=12, "浊度"=13, "叶绿素a"=14, "藻密度"=15, "蓝绿藻"=16, "氧化还原电位"=17, "溶解氧%"=18, "盐度"=19, "水中油"=20, "高锰酸盐指数"=21, "化学需氧量"=22, "比电导率"=23, "总溶解固体"=24, "pH电极电位"=25] ("下拉列表")
                  n136 = Bundle By Name(cluster=w283, "蓝绿藻"=1.0 ("DO")) -> (w282:T5)
                  n137 = call "多参数测量数据读取.vi"("探头选择"=w287) -> ("测量数据块"=w281:T6)  [unwired: 8 in, 2 out]
                  n138 = global write "多参数全局变量.vi" "蓝绿藻数据区"(w281) -> ()
                  n139 = call "多参数据转列表.vi"("参数名"="蓝绿藻", "测量数据块"=w281) -> ("添加的数组"=w280:string[][])  [unwired: 9 in]
                  n140 = Index Array(array=w280) -> (element #1=w279:string[], element #2=w278:string[])  [unwired: 4 in]
                  n141 = Insert Into Array(array=w286, new element=w278) -> (w285:string[][])  [unwired: 2 in]
                }
                frame 17 {
                  w298 = u16 17 items=["氨氮"=3, "水温"=9, "pH"=10, "溶解氧"=11, "电导率"=12, "浊度"=13, "叶绿素a"=14, "藻密度"=15, "蓝绿藻"=16, "氧化还原电位"=17, "溶解氧%"=18, "盐度"=19, "水中油"=20, "高锰酸盐指数"=21, "化学需氧量"=22, "比电导率"=23, "总溶解固体"=24, "pH电极电位"=25] ("下拉列表")
                  n142 = Bundle By Name(cluster=w294, "ORP"=1.0 ("DO")) -> (w293:T5)
                  n143 = call "多参数测量数据读取.vi"("探头选择"=w298) -> ("测量数据块"=w292:T6)  [unwired: 8 in, 2 out]
                  n144 = global write "多参数全局变量.vi" "ORP数据区"(w292) -> ()
                  n145 = call "多参数据转列表.vi"("参数名"="ORP", "测量数据块"=w292) -> ("添加的数组"=w291:string[][])  [unwired: 9 in]
                  n146 = Index Array(array=w291) -> (element #1=w290:string[], element #2=w288:string[])  [unwired: 4 in]
                  n147 = Insert Into Array(array=w297, new element=w288) -> (w296:string[][])  [unwired: 2 in]
                }
                frame 20 {
                  w307 = u16 20 items=["氨氮"=3, "水温"=9, "pH"=10, "溶解氧"=11, "电导率"=12, "浊度"=13, "叶绿素a"=14, "藻密度"=15, "蓝绿藻"=16, "氧化还原电位"=17, "溶解氧%"=18, "盐度"=19, "水中油"=20, "高锰酸盐指数"=21, "化学需氧量"=22, "比电导率"=23, "总溶解固体"=24, "pH电极电位"=25] ("下拉列表")
                  n148 = call "多参数测量数据读取.vi"("探头选择"=w307) -> ("测量数据块"=w303:T6)  [unwired: 8 in, 2 out]
                  n149 = call "多参数据转列表.vi"("参数名"="水中油", "测量数据块"=w303) -> ("添加的数组"=w301:string[][])  [unwired: 9 in]
                  n150 = Index Array(array=w301) -> (element #1=w300:string[], element #2=w299:string[])  [unwired: 4 in]
                  n151 = Insert Into Array(array=w306, new element=w299) -> (w305:string[][])  [unwired: 2 in]
                }
                frame 21 {
                  w316 = u16 21 items=["氨氮"=3, "水温"=9, "pH"=10, "溶解氧"=11, "电导率"=12, "浊度"=13, "叶绿素a"=14, "藻密度"=15, "蓝绿藻"=16, "氧化还原电位"=17, "溶解氧%"=18, "盐度"=19, "水中油"=20, "高锰酸盐指数"=21, "化学需氧量"=22, "比电导率"=23, "总溶解固体"=24, "pH电极电位"=25] ("下拉列表")
                  n152 = call "多参数测量数据读取.vi"("探头选择"=w316) -> ("测量数据块"=w312:T6)  [unwired: 8 in, 2 out]
                  n153 = call "多参数据转列表.vi"("参数名"="高锰酸盐指数", "测量数据块"=w312) -> ("添加的数组"=w311:string[][])  [unwired: 9 in]
                  n154 = Index Array(array=w311) -> (element #1=w309:string[], element #2=w308:string[])  [unwired: 4 in]
                  n155 = Insert Into Array(array=w315, new element=w308) -> (w314:string[][])  [unwired: 2 in]
                }
                frame 22 {
                  w325 = u16 22 items=["氨氮"=3, "水温"=9, "pH"=10, "溶解氧"=11, "电导率"=12, "浊度"=13, "叶绿素a"=14, "藻密度"=15, "蓝绿藻"=16, "氧化还原电位"=17, "溶解氧%"=18, "盐度"=19, "水中油"=20, "高锰酸盐指数"=21, "化学需氧量"=22, "比电导率"=23, "总溶解固体"=24, "pH电极电位"=25] ("下拉列表")
                  n156 = call "多参数测量数据读取.vi"("探头选择"=w325) -> ("测量数据块"=w321:T6)  [unwired: 8 in, 2 out]
                  n157 = call "多参数据转列表.vi"("参数名"="化学需氧量", "测量数据块"=w321) -> ("添加的数组"=w320:string[][])  [unwired: 9 in]
                  n158 = Index Array(array=w320) -> (element #1=w318:string[], element #2=w317:string[])  [unwired: 4 in]
                  n159 = Insert Into Array(array=w324, new element=w317) -> (w323:string[][])  [unwired: 2 in]
                }
              }
            }
            n160 = global write "多参数全局变量.vi" "传感器通道号"(w131) -> ()
            n161 = property on="数据区" class="MCListbox (严格)"("ColHdrString"=w137, "ItemNames"=w136) -> ()  [unwired: 2 in, 2 out]
          }
          frame Error {
          }
        }
      }
    }
  }
  n162 = property on="窗格" class="Pane"("Origin"=T2 {"Horizontal"=0, "Vertical"=0} ("原点")) -> ()  [unwired: 2 in, 2 out]
  n163 = call <vilib>:"Application Directory.vi"() -> ("Application Directory"=w2:path)
  n164 = Build Path(base path=w2, name or relative path="data\\sys.ini" ("名称或相对路径")) -> (appended path=w4:path)
  n165 = call <vilib>:"Open Config Data.vi"("configuration file path"=w4) -> ("error out"=w8:errorcluster, "refnum"=w5:T7)  [unwired: 8 in, 1 out]
  n166 = vi-ref "斯坦道仪器.lvlib:五参数水样测试.vi"() -> (w17:refnum<vi>)
  n167 = vi-ref "斯坦道仪器.lvlib:多参数断电保存全局变量.vi"() -> (w6:refnum<vi>)
  n168 = call <userlib>:"Read Panel from INI__ogtk.vi"("error in (no error)"=w8, "VI ref"=w6, "refnum"=w5) -> ("error out"=w9:errorcluster, "refnum out"=w7:T7)  [unwired: 7 in]
  n169 = property on="打开串口" class="Bool (严格)"("Val(Sgnl)"=TRUE ("值(信号)")) -> (error out=w10:errorcluster)  [unwired: 2 in, 1 out]
  n170 = call <vilib>:"Close Config Data.vi"("error in (no error)"=w9, "refnum"=w7) -> ("error out"=w1:errorcluster)  [unwired: 8 in, 1 out]
  n171 = Obtain Notifier(name (unnamed)="MPFlow" ("名称（未命名）"), notification data type=FALSE) -> (notifier out=w16:refnum<notifier>)  [unwired: 2 in, 2 out]
  n172 = control-ref of="控制命令区探头选择"() -> (w15:refnum<vi>)
  n173 = control-ref of="校准区探头选择"() -> (w12:refnum<vi>)
  n174 = control-ref of="K"() -> (w14:refnum<vi>)
  n175 = control-ref of="B"() -> (w13:refnum<vi>)
  n176 = while {
    tunnel: w17 -> [w331]
    tunnel: w16 -> [w330]
    tunnel: w15 -> [w329]
    tunnel: w14 -> [w328]
    tunnel: w13 -> [w327]
    tunnel: w12 -> [w326]
    tunnel: w10 -> [_]
    tunnel: w1 -> [_]
    stop <- FALSE stop-if-true
    n177 = event shown="[1] \"质控参数设置\": 值改变" {
      selector: _ -> [_ _ _ _ _ _ _ _ _ _ _ _ _ _ _ _ _ _ _ _ _]
      dyn-events: _ -> [_ _ _ _ _ _ _ _ _ _ _ _ _ _ _ _ _ _ _ _ _]
      timeout: _ -> [_ _ _ _ _ _ _ _ _ _ _ _ _ _ _ _ _ _ _ _ _]
      tunnel: w331 -> [_ _ _ _ w374 _ _ _ _ _ _ _ _ _ _ _ _ _ _ _ _]
      tunnel: w330 -> [_ _ _ _ _ w396 _ _ _ _ _ _ _ _ _ _ _ _ _ _ _]
      tunnel: w329 -> [_ _ _ _ _ _ _ _ _ _ _ _ _ _ _ _ w440 w447 _ _ _]
      tunnel: w328 -> [_ _ _ _ _ _ _ _ _ _ _ _ _ _ _ _ _ _ w453 _ _]
      tunnel: w327 -> [_ _ _ _ _ _ _ _ _ _ _ _ _ _ _ _ _ _ w455 _ _]
      tunnel: w326 -> [_ _ _ _ _ _ _ _ _ _ _ _ _ _ _ _ _ _ w457 _ w469]
      event Timeout {
        n178 = event-data() -> ()  [unwired: 1 in, 3 out]
      }
      event "质控参数设置": Value Change {
        n179 = event-data() -> ()  [unwired: 1 in, 6 out]
        n180 = global read "多参数断电保存全局变量.vi" "质控参数设置"() -> (w333:T10)
        n181 = call "多参数质控参数设置.vi"("质控参数设置"=w333) -> ("输出簇"=w334:T11)  [unwired: 10 in]
        n182 = Unbundle By Name(w334) -> ("确定"=w335:bool)
        n183 = case shown="真" w335 {
          tunnel: w334 -> [_ w337]
          tunnel: w333 -> [_ w336]
          frame False {
          }
          frame True {
            n184 = flat-sequence {
              tunnel: w337 -> [w345]
              tunnel: w336 -> [w344]
              frame #0 {
                n185 = Unbundle By Name(w345) -> ("水温标准液标准浓度"=w343:dbl, "酸碱度标准液标准浓度"=w342:dbl, "溶解氧标准液标准浓度"=w341:dbl, "电导率标准液标准浓度"=w340:dbl, "浊度标准液标准浓度"=w339:dbl)
                n186 = Bundle By Name(cluster=w344, "水温标准液标准浓度"=w343, "酸碱度标准液标准浓度"=w342, "溶解氧标准液标准浓度"=w341, "电导率标准液标准浓度"=w340, "浊度标准液标准浓度"=w339) -> (w338:T10)
                n187 = global write "多参数断电保存全局变量.vi" "质控参数设置"(w338) -> ()
              }
              frame #1 {
                n188 = call <vilib>:"Application Directory.vi"() -> ("Application Directory"=w359:path)
                n189 = Build Path(base path=w359, name or relative path="data\\sys.ini" ("名称或相对路径")) -> (appended path=w357:path)
                n190 = call <vilib>:"Open Config Data.vi"("configuration file path"=w357) -> ("error out"=w353:errorcluster, "refnum"=w356:T7)  [unwired: 8 in, 1 out]
                n191 = vi-ref "斯坦道仪器.lvlib:多参数断电保存全局变量.vi"() -> (w355:refnum<vi>)
                n192 = call <userlib>:"Write Panel to INI__ogtk.vi"("error in (no error)"=w353, "VI ref"=w355, "refnum"=w356) -> ("error out"=w352:errorcluster, "refnum out"=w354:T7)  [unwired: 7 in]
                n193 = call <vilib>:"Close Config Data.vi"("error in (no error)"=w352, "refnum"=w354) -> ("error out"=w347:errorcluster, "file path"=w346:path)  [unwired: 8 in]
                n194 = Open/Create/Replace File(file path (use dialog)=w346, error in=w347) -> (refnum out=w350:refnum<file>, error out=w351:errorcluster)  [unwired: 4 in, 1 out]
                n195 = Flush File(refnum=w350, error in=w351) -> (refnum out=w349:refnum<file>, error out=w348:errorcluster)
                n196 = Close File(refnum=w349, error in=w348) -> ()  [unwired: 2 out]
              }
            }
          }
        }
      }
      event "释放串口": Value Change {
        n197 = event-data() -> ("NewVal"=w360:bool)  [unwired: 1 in, 5 out]
        n198 = case shown="真" w360 {
          frame False {
          }
          frame True {
            n199 = call "多参数通讯.vi"("STEP"=enum16{"open", "read", "write", "close"}."close") -> ("error out"=w361:errorcluster)  [unwired: 8 in, 2 out]
            n200 = case shown="无错误" w361 {
              frame No Error {
                n201 = property on="打开串口" class="Bool (严格)"("DisabledEnum"=T8."Enabled" ("禁用")) -> ()  [unwired: 2 in, 2 out]
              }
              frame Error {
              }
            }
          }
        }
      }
      event "打开串口": Value Change {
        n202 = event-data() -> ("NewVal"=w364:bool)  [unwired: 1 in, 5 out]
        n203 = case shown="真" w364 {
          frame False {
          }
          frame True {
            n204 = call "多参数通讯.vi"("STEP"=enum16{"open", "read", "write", "close"}."open") -> ("error out"=w365:errorcluster)  [unwired: 8 in, 2 out]
            n205 = case shown="错误" w365 {
              tunnel: [T8."Disabled and Grayed Out" ("禁用") T8."Enabled" ("禁用")] -> w367
              frame No Error {
              }
              frame Error {
                n206 = One Button Dialog(message="多参数串口打开失败" ("消息")) -> ()  [unwired: 1 in, 1 out]
              }
            }
            n207 = property on="打开串口" class="Bool (严格)"("DisabledEnum"=w367, "Value"=FALSE ("打开串口")) -> ()  [unwired: 2 in, 2 out]
          }
        }
      }
      event "手动启动": Value Change {
        n208 = event-data() -> ()  [unwired: 1 in, 6 out]
        n209 = call "多参数启动参数对话框.vi"() -> ("确认"=w373:bool, "测量时间"=w372:dbl)  [unwired: 10 in]
        n210 = case shown="真" w373 {
          tunnel: w374 -> [_ w376]
          tunnel: w372 -> [_ w375]
          frame False {
          }
          frame True {
            n211 = property class="VI"(reference=w376) -> ("Name"=w380:string, "Exec.State"=w378:T12)  [unwired: 1 in, 2 out]
            n212 = Open VI Reference(type specifier VI Refnum (for type only)=refnum<vi> refnum ("类型说明符VI引用句柄（仅用于类型）"), vi path=w380, options=128 ("选项")) -> (vi reference=w379:refnum<vi>)  [unwired: 3 in, 1 out]
            n213 = case shown="\"Idle\"" w378 {
              tunnel: w379 -> [w384 w391]
              tunnel: [w384 w390] -> w377
              tunnel: w375 -> [_ w385]
              frame "Bad", Default {
                n214 = One Button Dialog(message="仪器已经启动，无需重复启动" ("消息")) -> ()  [unwired: 1 in, 1 out]
              }
              frame "Idle" {
                n215 = global read "系统变量.vi" "运行模式"() -> (w387:enum16{"维护模式", "常规模式", "应急模式", "质控模式"})
                n216 = case shown="\"常规模式\", 默认" w387 {
                  tunnel: ["M" ("数据标记表") "hd" ("数据标记表")] -> w386
                  frame "维护模式" {
                  }
                  frame "常规模式", Default {
                  }
                }
                n217 = Bundle By Name(cluster=T9 {"测量模式"=enum."水样测试", "数据标记表"="", "测量时间"=0.0} ("启动参数"), "数据标记表"=w386, "测量时间"=w385) -> (w388:T9)
                n218 = call-by-ref "开始异步调用"(reference=w391, "启动参数"=w388) -> (reference out=w390:refnum<vi>)  [unwired: 12 in, 1 out]
              }
            }
            n219 = Close Reference(reference=w377) -> ()  [unwired: 1 in, 1 out]
          }
        }
      }
      event "停止": Value Change {
        n220 = event-data() -> ()  [unwired: 1 in, 6 out]
        n221 = Two Button Dialog(message="请再一次确认是否停止测量" ("消息")) -> (T button?=w394:bool)  [unwired: 2 in]
        n222 = case shown="真" w394 {
          tunnel: w396 -> [_ w399]
          frame False {
          }
          frame True {
            w397 = u16 11 items=["启动测量（全部）"=1, "初始化（清洗）"=10, "停止测量（全部）"=11, "校时"=13, "启动测量（单个传感器）"=19, "停止测量（单个传感器）"=20] ("控制命令")
            w398 = u16 10 items=["氨氮"=3, "水温"=9, "pH值"=10, "溶解氧"=11, "电导率"=12, "浊度"=13, "叶绿素a"=14, "藻密度"=15, "蓝绿藻"=16, "氧化还原电位"=17, "溶解氧%"=18, "盐度"=19] ("站号")
            n223 = Send Notification(notification=TRUE ("通知"), notifier=w399) -> ()  [unwired: 1 in, 2 out]
            n224 = call "多参数控制命令.vi"("控制命令"=w397, "站号"=w398) -> ()  [unwired: 9 in, 1 out]
          }
        }
      }
      event "设置": Value Change {
        n225 = event-data() -> ()  [unwired: 1 in, 6 out]
        n226 = property on="窗格" class="Pane"("Origin"=T2 {"Horizontal"=0, "Vertical"=628} ("原点")) -> ()  [unwired: 2 in, 2 out]
      }
      event "返回": Value Change {
        n227 = event-data() -> ()  [unwired: 1 in, 6 out]
        n228 = property on="窗格" class="Pane"("Origin"=T2 {"Horizontal"=0, "Vertical"=0} ("原点")) -> ()  [unwired: 2 in, 2 out]
      }
      event "传感器参数读取": Value Change {
        n229 = event-data() -> ()  [unwired: 1 in, 6 out]
        n230 = call "多参数传感器参数读取.vi"() -> ("error out"=w403:errorcluster, "添加的数组"=w404:string[][])  [unwired: 10 in]
        n231 = call <vilib>:"General Error Handler.vi"("error in (no error)"=w403) -> ()  [unwired: 10 in, 5 out]
        n232 = property on="传感器区" class="MCListbox (严格)"("ItemNames"=w404) -> ()  [unwired: 2 in, 2 out]
      }
      event "关键参数区读取": Value Change {
        n233 = event-data() -> ()  [unwired: 1 in, 6 out]
        n234 = call "多参数关键参数读取.vi"() -> ("error out"=w405:errorcluster, "添加的数组"=w406:string[][])  [unwired: 10 in]
        n235 = call <vilib>:"General Error Handler.vi"("error in (no error)"=w405) -> ()  [unwired: 10 in, 5 out]
        n236 = property on="关键参数区" class="MCListbox (严格)"("ItemNames"=w406) -> ()  [unwired: 2 in, 2 out]
      }
      event "测量数据区读取": Value Change {
        n237 = event-data() -> ()  [unwired: 1 in, 6 out]
        n238 = call "多参数测量数据读取.vi"("探头选择"="探头选择") -> ("error out"=w409:errorcluster, "添加的数组"=w407:string[][])  [unwired: 8 in, 1 out]
        n239 = call <vilib>:"General Error Handler.vi"("error in (no error)"=w409) -> ()  [unwired: 10 in, 5 out]
        n240 = property on="测量数据区" class="MCListbox (严格)"("ItemNames"=w407) -> ()  [unwired: 2 in, 2 out]
      }
      event "状态告警区读取": Value Change {
        n241 = event-data() -> ()  [unwired: 1 in, 6 out]
        n242 = call "多参数状态告警区读取.vi"() -> ("error out"=w410:errorcluster, "添加的数组"=w411:string[][])  [unwired: 9 in, 1 out]
        n243 = call <vilib>:"General Error Handler.vi"("error in (no error)"=w410) -> ()  [unwired: 10 in, 5 out]
        n244 = property on="状态告警区" class="MCListbox (严格)"("ItemNames"=w411) -> ()  [unwired: 2 in, 2 out]
      }
      event "同步时间": Value Change {
        w412 = u16 13 items=["启动测量（全部）"=1, "初始化（清洗）"=10, "停止测量（全部）"=11, "校时"=13, "启动测量（单个传感器）"=19, "停止测量（单个传感器）"=20] ("控制命令")
        w413 = u16 9 items=["氨氮"=3, "水温"=9, "pH值"=10, "溶解氧"=11, "电导率"=12, "浊度"=13, "叶绿素a"=14, "藻密度"=15, "蓝绿藻"=16, "氧化还原电位"=17, "溶解氧%"=18, "盐度"=19] ("站号")
        n245 = event-data() -> ()  [unwired: 1 in, 6 out]
        n246 = call "多参数控制命令.vi"("控制命令"=w412, "站号"=w413) -> ("error out"=w415:errorcluster)  [unwired: 9 in]
        n247 = case shown="错误" w415 {
          tunnel: ["时间同步成功" ("消息") "时间同步失败" ("消息")] -> w414
          frame No Error {
          }
          frame Error {
          }
        }
        n248 = One Button Dialog(message=w414) -> ()  [unwired: 1 in, 1 out]
      }
      event "启动测量(全部)": Value Change {
        w418 = u16 1 items=["启动测量（全部）"=1, "初始化（清洗）"=10, "停止测量（全部）"=11, "校时"=13, "启动测量（单个传感器）"=19, "停止测量（单个传感器）"=20] ("控制命令")
        w419 = u16 9 items=["氨氮"=3, "水温"=9, "pH值"=10, "溶解氧"=11, "电导率"=12, "浊度"=13, "叶绿素a"=14, "藻密度"=15, "蓝绿藻"=16, "氧化还原电位"=17, "溶解氧%"=18, "盐度"=19] ("站号")
        n249 = event-data() -> ()  [unwired: 1 in, 6 out]
        n250 = call "多参数控制命令.vi"("控制命令"=w418, "站号"=w419) -> ("error out"=w421:errorcluster)  [unwired: 9 in]
        n251 = case shown="无错误" w421 {
          tunnel: ["启动成功" ("消息") "启动失败" ("消息")] -> w420
          frame No Error {
          }
          frame Error {
          }
        }
        n252 = One Button Dialog(message=w420) -> ()  [unwired: 1 in, 1 out]
      }
      event "停止测量(全部)": Value Change {
        w426 = u16 11 items=["启动测量（全部）"=1, "初始化（清洗）"=10, "停止测量（全部）"=11, "校时"=13, "启动测量（单个传感器）"=19, "停止测量（单个传感器）"=20] ("控制命令")
        w427 = u16 9 items=["氨氮"=3, "水温"=9, "pH值"=10, "溶解氧"=11, "电导率"=12, "浊度"=13, "叶绿素a"=14, "藻密度"=15, "蓝绿藻"=16, "氧化还原电位"=17, "溶解氧%"=18, "盐度"=19] ("站号")
        n253 = event-data() -> ()  [unwired: 1 in, 6 out]
        n254 = call "多参数控制命令.vi"("控制命令"=w426, "站号"=w427) -> ("error out"=w425:errorcluster)  [unwired: 9 in]
        n255 = case shown="错误" w425 {
          tunnel: ["停止成功" ("消息") "停止失败" ("消息")] -> w424
          frame No Error {
          }
          frame Error {
          }
        }
        n256 = One Button Dialog(message=w424) -> ()  [unwired: 1 in, 1 out]
      }
      event "初始化(清洗)": Value Change {
        w432 = u16 10 items=["启动测量（全部）"=1, "初始化（清洗）"=10, "停止测量（全部）"=11, "校时"=13, "启动测量（单个传感器）"=19, "停止测量（单个传感器）"=20] ("控制命令")
        w433 = u16 9 items=["氨氮"=3, "水温"=9, "pH值"=10, "溶解氧"=11, "电导率"=12, "浊度"=13, "叶绿素a"=14, "藻密度"=15, "蓝绿藻"=16, "氧化还原电位"=17, "溶解氧%"=18, "盐度"=19] ("站号")
        n257 = event-data() -> ()  [unwired: 1 in, 6 out]
        n258 = call "多参数控制命令.vi"("控制命令"=w432, "站号"=w433) -> ("error out"=w430:errorcluster)  [unwired: 9 in]
        n259 = case shown="错误" w430 {
          tunnel: ["初始化成功" ("消息") "初始化失败" ("消息")] -> w431
          frame No Error {
          }
          frame Error {
          }
        }
        n260 = One Button Dialog(message=w431) -> ()  [unwired: 1 in, 1 out]
      }
      event "启动测量(单探)": Value Change {
        w436 = u16 19 items=["启动测量（全部）"=1, "初始化（清洗）"=10, "停止测量（全部）"=11, "校时"=13, "启动测量（单个传感器）"=19, "停止测量（单个传感器）"=20] ("控制命令")
        n261 = event-data() -> ()  [unwired: 1 in, 6 out]
        n262 = property class="Ring (严格)"(reference=w440) -> ("Value"=w439:u16)  [unwired: 1 in, 2 out]
        n263 = call "多参数控制命令.vi"("控制命令"=w436, "站号"=w439) -> ("error out"=w438:errorcluster)  [unwired: 9 in]
        n264 = case shown="无错误" w438 {
          tunnel: ["启动成功" ("消息") "启动失败" ("消息")] -> w437
          frame No Error {
          }
          frame Error {
          }
        }
        n265 = One Button Dialog(message=w437) -> ()  [unwired: 1 in, 1 out]
      }
      event "停止测量(单探)": Value Change {
        w443 = u16 20 items=["启动测量（全部）"=1, "初始化（清洗）"=10, "停止测量（全部）"=11, "校时"=13, "启动测量（单个传感器）"=19, "停止测量（单个传感器）"=20] ("控制命令")
        n266 = event-data() -> ()  [unwired: 1 in, 6 out]
        n267 = property class="Ring (严格)"(reference=w447) -> ("Value"=w446:u16)  [unwired: 1 in, 2 out]
        n268 = call "多参数控制命令.vi"("控制命令"=w443, "站号"=w446) -> ("error out"=w445:errorcluster)  [unwired: 9 in]
        n269 = case shown="错误" w445 {
          tunnel: ["停止成功" ("消息") "停止失败" ("消息")] -> w444
          frame No Error {
          }
          frame Error {
          }
        }
        n270 = One Button Dialog(message=w444) -> ()  [unwired: 1 in, 1 out]
      }
      event "写入KB": Value Change {
        n271 = event-data() -> ()  [unwired: 1 in, 6 out]
        n272 = property class="DigNum (严格)"(reference=w453) -> ("Value"=w452:dbl)  [unwired: 1 in, 2 out]
        n273 = property class="DigNum (严格)"(reference=w455) -> ("Value"=w454:dbl)  [unwired: 1 in, 2 out]
        n274 = property class="Ring (严格)"(reference=w457) -> ("Value"=w456:u16)  [unwired: 1 in, 2 out]
        n275 = call "多参数校准写入.vi"("B"=w454, "K"=w452, "站号"=w456) -> ("error out"=w450:errorcluster)  [unwired: 8 in]
        n276 = case shown="错误" w450 {
          tunnel: ["写入成功" ("消息") "写入失败" ("消息")] -> w451
          frame No Error {
          }
          frame Error {
          }
        }
        n277 = One Button Dialog(message=w451) -> ()  [unwired: 1 in, 1 out]
      }
      event "K", "B": Mouse Down {
        n278 = event-data() -> ("CtlRef"=w463:refnum<vi>)  [unwired: 1 in, 5 out]
        n279 = property class="DigNum (严格)"(reference=w463) -> (reference out=w462:refnum<vi>, "Value"=w461:dbl)  [unwired: 1 in, 1 out]
        n280 = call "数字键盘.vi"("OldNumber"=w461) -> ("NewNumber"=w460:dbl)
        n281 = property class="DigNum (严格)"(reference=w462, "Value"=w460) -> ()  [unwired: 1 in, 2 out]
      }
      event "读取KB": Value Change {
        n282 = event-data() -> ()  [unwired: 1 in, 6 out]
        n283 = property class="Ring (严格)"(reference=w469) -> ("Value"=w468:u16)  [unwired: 1 in, 2 out]
        n284 = call "多参校准读取.vi"("站号"=w468) -> ("error out"=w464:errorcluster, "B"=→"B":dbl, "K"=→"K":dbl)  [unwired: 8 in]
        n285 = case shown="无错误" w464 {
          tunnel: ["读取成功" ("消息") "读取失败" ("消息")] -> w465
          frame No Error {
          }
          frame Error {
          }
        }
        n286 = One Button Dialog(message=w465) -> ()  [unwired: 1 in, 1 out]
      }
    }
  }
